vi "发送XBOX_Control_Msg.vi"(7 "消息优先级（正常）":T14=enum."Normal", 8 "error in (no error)":cluster{"状态":bool, "代码":i32, "源":string} caption="错误输入（无错误）", 10 "XBOX_Control":T1, 11 "消息待入队列":refnum<class "Message Enqueuer.lvclass">) -> (0 "error out":cluster{"状态":bool, "代码":i32, "源":string} caption="错误输出", 3 "消息待入队列输出":refnum<class "Message Enqueuer.lvclass">)   [LabVIEW 2014, in "ControlPanel.lvlib" / "XBOX_Control_Msg消息.lvclass"]
doc: "本VI将消息发送至操作者。"
uses:
  <vilib>/ActorFramework/Message Enqueuer/Message Enqueuer.lvclass
  <vilib>/ActorFramework/Message Enqueuer/Message Priority.ctl
  ctl/XBOX_Control.ctl
  <vilib>/MakerHub/Xbox-One-Controller/Private/Type Defs/Indicators/All Buttons Visual.ctl
  <vilib>/MakerHub/Xbox-One-Controller/Private/Type Defs/Indicators/A.ctl
  <vilib>/MakerHub/Xbox-One-Controller/Private/Type Defs/Indicators/B.ctl
  <vilib>/MakerHub/Xbox-One-Controller/Private/Type Defs/Indicators/X.ctl
  <vilib>/MakerHub/Xbox-One-Controller/Private/Type Defs/Indicators/Y.ctl
  <vilib>/MakerHub/Xbox-One-Controller/Private/Type Defs/Indicators/Left Bumper.ctl
  <vilib>/MakerHub/Xbox-One-Controller/Private/Type Defs/Indicators/Right Bumper.ctl
  <vilib>/MakerHub/Xbox-One-Controller/Private/Type Defs/Indicators/View.ctl
  <vilib>/MakerHub/Xbox-One-Controller/Private/Type Defs/Indicators/Menu.ctl
  <vilib>/MakerHub/Xbox-One-Controller/Private/Type Defs/Indicators/Thumbstick.ctl
  <vilib>/MakerHub/Xbox-One-Controller/Private/Type Defs/Indicators/All Axis Data.ctl
  <vilib>/MakerHub/Xbox-One-Controller/Private/Type Defs/Indicators/DPad Enum.ctl
  <vilib>/ActorFramework/Message Enqueuer/Message Enqueuer.lvclass/Message Enqueuer.ctl
  <vilib>/ActorFramework/Message Priority Queue/Priority Enqueue.vi
  <vilib>/MakerHub/Xbox-One-Controller/LMH-Xbox-One-Controller.lvlib
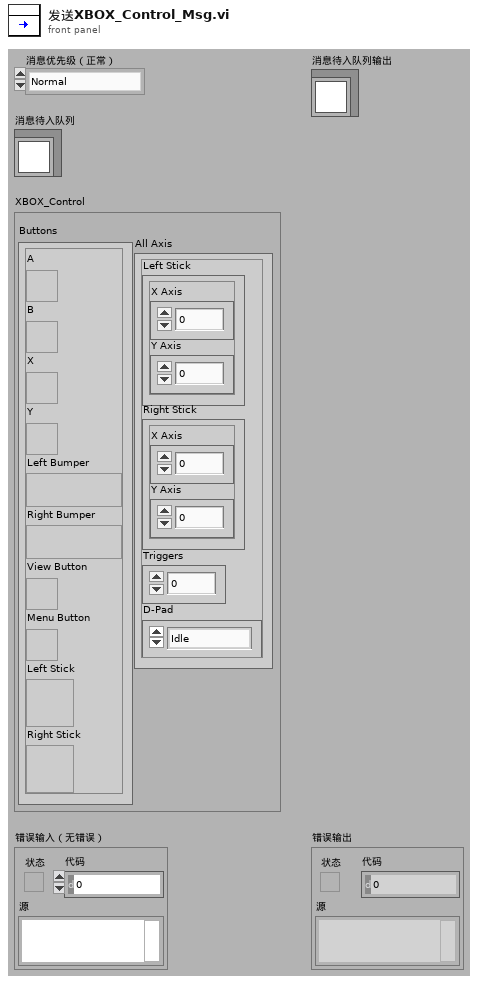
[diagram p1: front panel]
types:
  T1 = typedef "XBOX_Control.ctl" = cluster{"Buttons":T2, "All Axis":T12}
  T2 = typedef "LMH-Xbox-One-Controller.lvlib/All Buttons Visual.ctl" = cluster{"A":T3, "B":T4, "X":T5, "Y":T6, "Left Bumper":T7, "Right Bumper":T8, "View Button":T9, "Menu Button":T10, "Left Stick":T11, "Right Stick":T11}
  T3 = typedef "LMH-Xbox-One-Controller.lvlib/A.ctl" = bool
  T4 = typedef "LMH-Xbox-One-Controller.lvlib/B.ctl" = bool
  T5 = typedef "LMH-Xbox-One-Controller.lvlib/X.ctl" = bool
  T6 = typedef "LMH-Xbox-One-Controller.lvlib/Y.ctl" = bool
  T7 = typedef "LMH-Xbox-One-Controller.lvlib/Left Bumper.ctl" = bool
  T8 = typedef "LMH-Xbox-One-Controller.lvlib/Right Bumper.ctl" = bool
  T9 = typedef "LMH-Xbox-One-Controller.lvlib/View.ctl" = bool
  T10 = typedef "LMH-Xbox-One-Controller.lvlib/Menu.ctl" = bool
  T11 = typedef "LMH-Xbox-One-Controller.lvlib/Thumbstick.ctl" = bool
  T12 = typedef "LMH-Xbox-One-Controller.lvlib/All Axis Data.ctl" = cluster{"Left Stick":cluster{"X Axis":i32, "Y Axis":i32}, "Right Stick":cluster{"X Axis":i32, "Y Axis":i32}, "Triggers":i32, "D-Pad":T13}
  T13 = typedef "LMH-Xbox-One-Controller.lvlib/DPad Enum.ctl" = enum16{"Idle", "Up", "Up / Right", "Right", "Down / Right", "Down", "Down / Left", "Left", "Up / Left"}
  T14 = typedef "Actor Framework.lvlib/Message Enqueuer.lvclass/Message Priority.ctl" = enum16{"Low", "Normal", "High"}
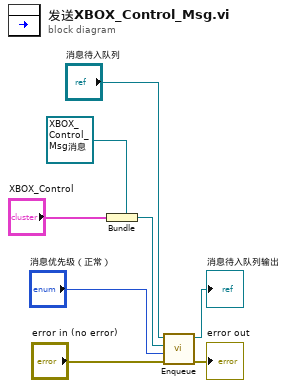
[diagram p0: block diagram]
diagram:
  n1 = Bundle(cluster=refnum<class "XBOX_Control_Msg消息.lvclass"> refnum ("Object"), "XBOX_Control") -> (w4:refnum<class "XBOX_Control_Msg消息.lvclass">)
  n2 = call <vilib>:"Enqueue.vi"("error in (no error)"="error in (no error)", "Message Priority (Normal)"="消息优先级（正常）", "Message"=w4, "Message Enqueuer in"="消息待入队列") -> ("error out"=→"error out":errorcluster, "Message Enqueuer out"=→"消息待入队列输出":refnum<class "Message Enqueuer.lvclass">)  [unwired: 6 in]
